vi "Periodic Tasks.vi"(8 "error in":errorcluster) -> ()   [LabVIEW 2015]
doc: "This VI runs in parallel to other tasks. It can contain as many user-defined periodic loops as you need. These can carry out PID or other sorts of timed response."
uses:
  LowGoalState.ctl
  SonarAction.ctl
  Example_Code/PressureSensor/PressureSensorAction.ctl
  RefnameEnum.ctl
  ServoAction.ctl
  TankDriveAction.ctl
  AutoAlignMode.ctl
  LEDSaction.ctl
  CatchAction.ctl
  CollectorWrapAction.ctl
  ShooterWrapperAction.ctl
  CollectorAction.ctl
  DoubleSolenoidAction.ctl
  SingleSolenoidAction.ctl
  <vilib>/Rock Robotics/SystemInterfaces/Utilities/FPGA_UtilitiesLED Source.ctl
  <vilib>/Rock Robotics/SystemInterfaces/Utilities/FPGA_UtilitiesLED State.ctl
  Robot Global Data.vi
  ArcadeDrivePieceWise.vi
  <vilib>/Rock Robotics/WPI/Compressor/WPI_CompressorGetSetRefNum.vi
  PassState.ctl
panel:
  in  "ShooterWait":i32=750
  in  "ShooterPassWait":i32
  in  "CutoffPressure":dbl=70.0
  out "LowGoalShotTimer":u32=50
  out "LowGoalShotIterations":i32=2744
  in  "PiecewiseCutoff":dbl=0.7 format="%#_13g"
  in  "ArcadeDeadzone":dbl=0.05 format="%#_13g"
  out "PassTimer":u32
  out "PassIterations":i32
  out "ServoTimer":u32
  out "ServoIterations":i32
  in  "HalfDriveScaler":dbl=0.7 min=0.0 max=1.0 step=0.05 format="%#_13g"
  out "ElevatedPassTimer":u32=50
  out "ElevatedPassIterations":i32=2744
  out "GroundPassTimer":u32=50
  out "GroundWrapperIterations":i32=2743
  out "PressureSensorTimer":u32
  out "PressureSensorIterations":i32
  out "AutoDistanceIterations":i32=6512
  out "AutoDistanceTimer":u32=20
  in  "Slowdown":dbl=12.0 format="%#_13g"
  in  "Brake":dbl=6.0 format="%#_13g"
  in  "DesiredDistance":dbl=144.0 format="%#_13g"
  out "CatcherWrapperIterations":i32=2744
  out "CatcherWrapperTimer":u32=50
  out "CollectorWrapperTimer":u32=50
  out "CollectorWrapperIterations":i32=2743
  out "ShooterWrapperIterations":i32=2667
  out "ShooterWrapperTimer":u32=50
  out "CollectorIterations":i32=2737
  out "ClapperIterations":i32=2743
  out "RollerPneumaticIterations":i32=2743
  out "RollerMotorIterations":i32=2742
  out "FiringCylinderIterations":i32=2745
  out "KickerIterations":i32=2744
  out "SonicShifterIterations":i32=2744
  out "TankDriveIterations":i32=6485
  out "Collector Timer":u32=50
  out "Clapper Timer":u32=50
  out "Roller Pneumatic Timer":u32=50
  out "Firing Cylinder Timer":u32=50
  out "Sonic Shifter Timer":u32=50
  out "Kicker Timer":u32=50
  out "Roller Motor Timer":u32=51
  out "Tank Drive Timer":u32=21
  # "ARCADE"
  # "CATCH"
  # "SHOOTER WRAP"
  # "SONIC SHIFTER"
  # "TANK DRIVE"
  # "KICKER"
  # "PRESSURE SENSOR"
  # "COLLECTOR WRAP"
  # "COLLECTOR ARM"
  # "ROLLER MOTOR"
  # "SERVO"
  # "FIRING CYLINDERS"
  # "AUTODISTANCE"
  # "ROLLER PNEUMATIC"
  # "CLAPPER"
  # "ELEVATED PASS"
  # "GROUND PASS"
  # "COMBINED PASS"
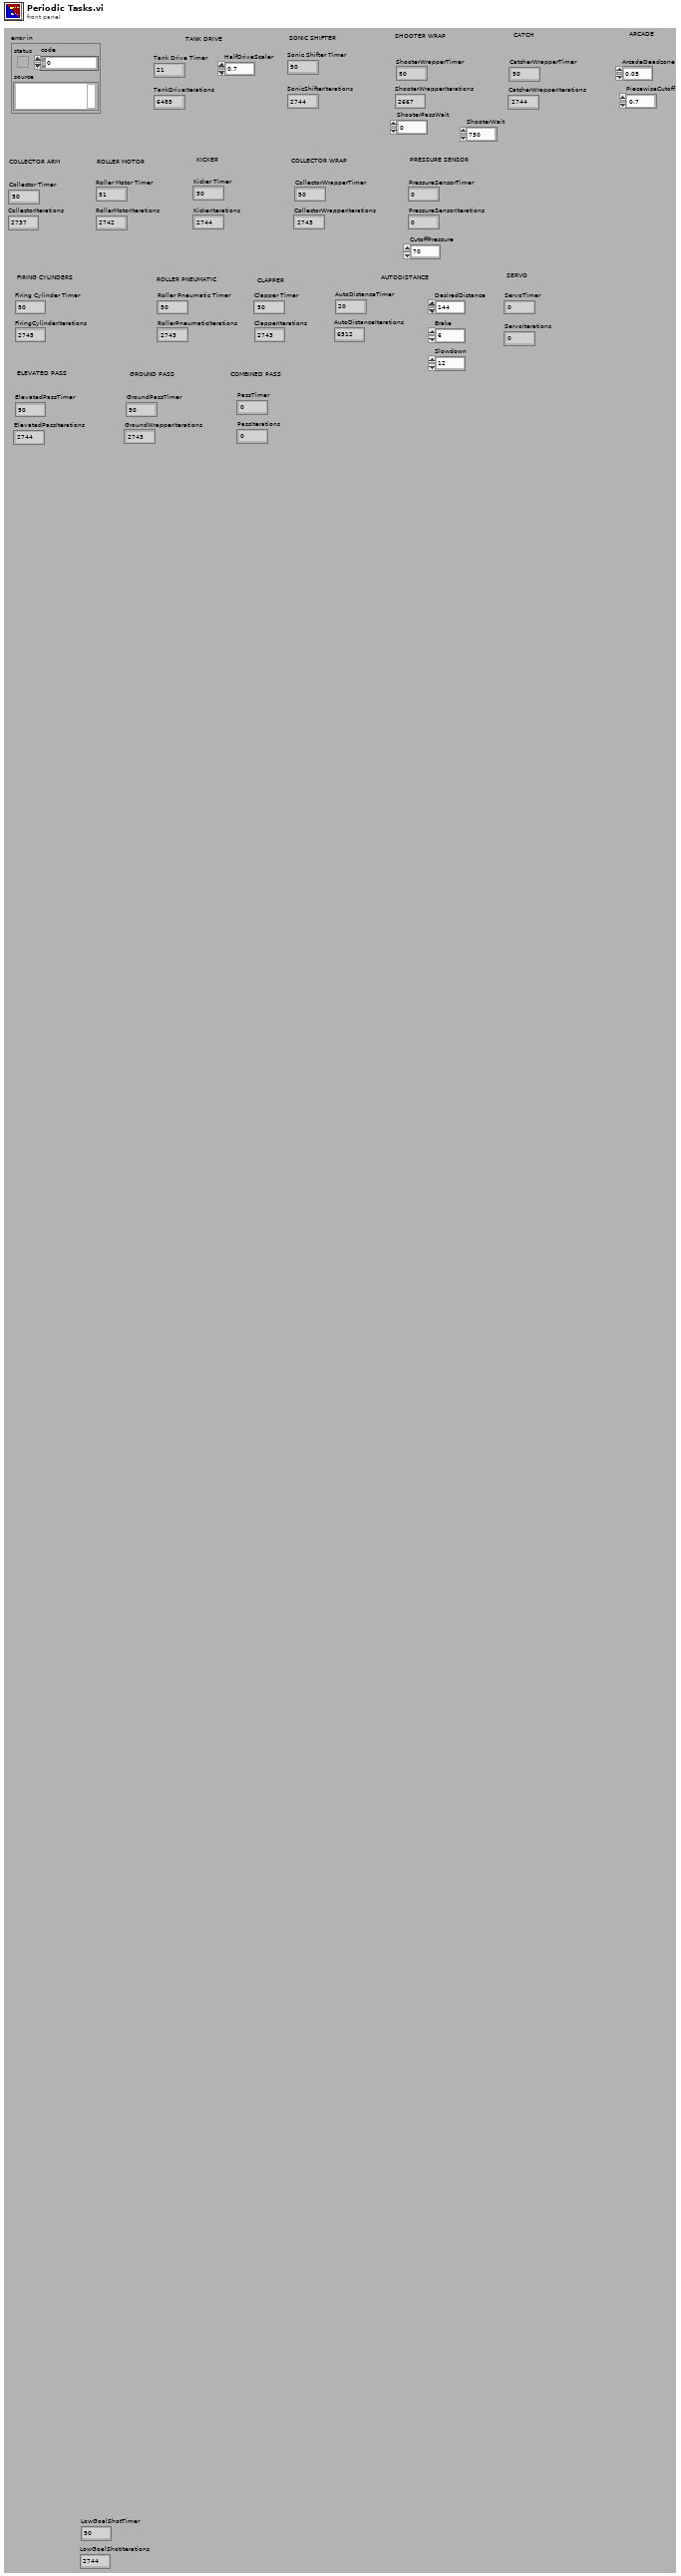
[diagram p1: front panel]
types:
  T1 = typedef "ShooterWrapperAction.ctl" = enum16{"Init", "CollectorDown", "CollectorUp"}
  T2 = typedef "CatchAction.ctl" = enum16{"Stop", "PreCatch", "Catch"}
  T3 = typedef "DoubleSolenoidAction.ctl" = enum16{"Init", "Middle", "In", "Out"}
  T4 = typedef "CollectorWrapAction.ctl" = enum16{"Stop", "PreCollect", "Collect"}
  T5 = typedef "SingleSolenoidAction.ctl" = enum16{"Init", "SetState", "Disable"}
  T6 = typedef "CollectorAction.ctl" = enum16{"Init", "Raise", "Lower", "Stop", "GetStatus"}
  T7 = typedef "FPGA_UtilitiesLED State.ctl" = enum16{"Off", "On", "Toggle"}
  T8 = typedef "FPGA_UtilitiesLED Source.ctl" = enum16{"User LED", "FPGA LED"}
  T9 = typedef "RefnameEnum.ctl" = enum16{"TankDrive", "Controller1", "Controller2", "SonicShifter", "Compressor"}
  T10 = typedef "WPI_CompressorDevRef.ctl" = cluster{"DevStatus":errorcluster, "DigitalInputDevRef":T11, "RelayDevRef":T14}
  T11 = typedef "WPI_DigitalInputDevRef.ctl" = cluster{"DevStatus":errorcluster, "DIO Channel":T12, "Digital Module":T13}
  T12 = typedef "FPGA_DIOChannel.ctl" = enum8{"DIO 1", "DIO 2", "DIO 3", "DIO 4", "DIO 5", "DIO 6", "DIO 7", "DIO 8", "DIO 9", "DIO 10", "DIO 11", "DIO 12", "DIO 13", "DIO 14", "Invalid"}
  T13 = typedef "FPGA_TypedefDigitalModule.ctl" = enum16{"Digital Module 1", "Digital Module 2"}
  T14 = typedef "WPI_RelayDevRef.ctl" = cluster{"DevStatus":errorcluster, "Relay Channel":T15, "Digital Module":T13, "Relay Direction":T16}
  T15 = typedef "FPGA_DIORelayChannel.ctl" = enum8{"Relay 1", "Relay 2", "Relay 3", "Relay 4", "Relay 5", "Relay 6", "Relay 7", "Relay 8", "Invalid"}
  T16 = typedef "WPI_RelayDirection.ctl" = enum16{"Both directions", "Forward only", "Reverse only"}
  T17 = typedef "RollerAction.ctl" = enum16{"Init", "Off", "Forward", "Reverse"}
  T18 = typedef "TankDriveAction.ctl" = enum16{"Init", "LinearDrive", "SetValue", "Disable"}
  T19 = typedef "SonarAction.ctl" = enum16{"Init", "ReadValue", "Disable"}
  T20 = typedef "AutoAlignMode.ctl" = enum16{"Fullspeed", "Linear"}
  T21 = typedef "PressureSensorAction.ctl" = enum16{"Init", "ReadValue", "Disable"}
  T22 = typedef "LEDSaction.ctl" = enum16{"Init", "10SecondsLeft", "LimitDown", "LimitUp", "CollectDown", "CollectUp", "NotHot", "Hot", "Shift", "RollBack", "RollFwd", "Shoot", "Distance Low", "DistanceHigh", "PressureLow", "PressureHigh"}
  T23 = typedef "PassState.ctl" = enum16{"Stop", "Pass"}
  T24 = typedef "ServoAction.ctl" = enum16{"Init", "SetAngle", "GetAngle", "Lower", "Raise", "Disable"}
  T25 = typedef "PassType.ctl" = enum16{"Ground", "Elevated"}
  T26 = typedef "LowGoalState.ctl" = enum16{"Stop", "Shoot"}
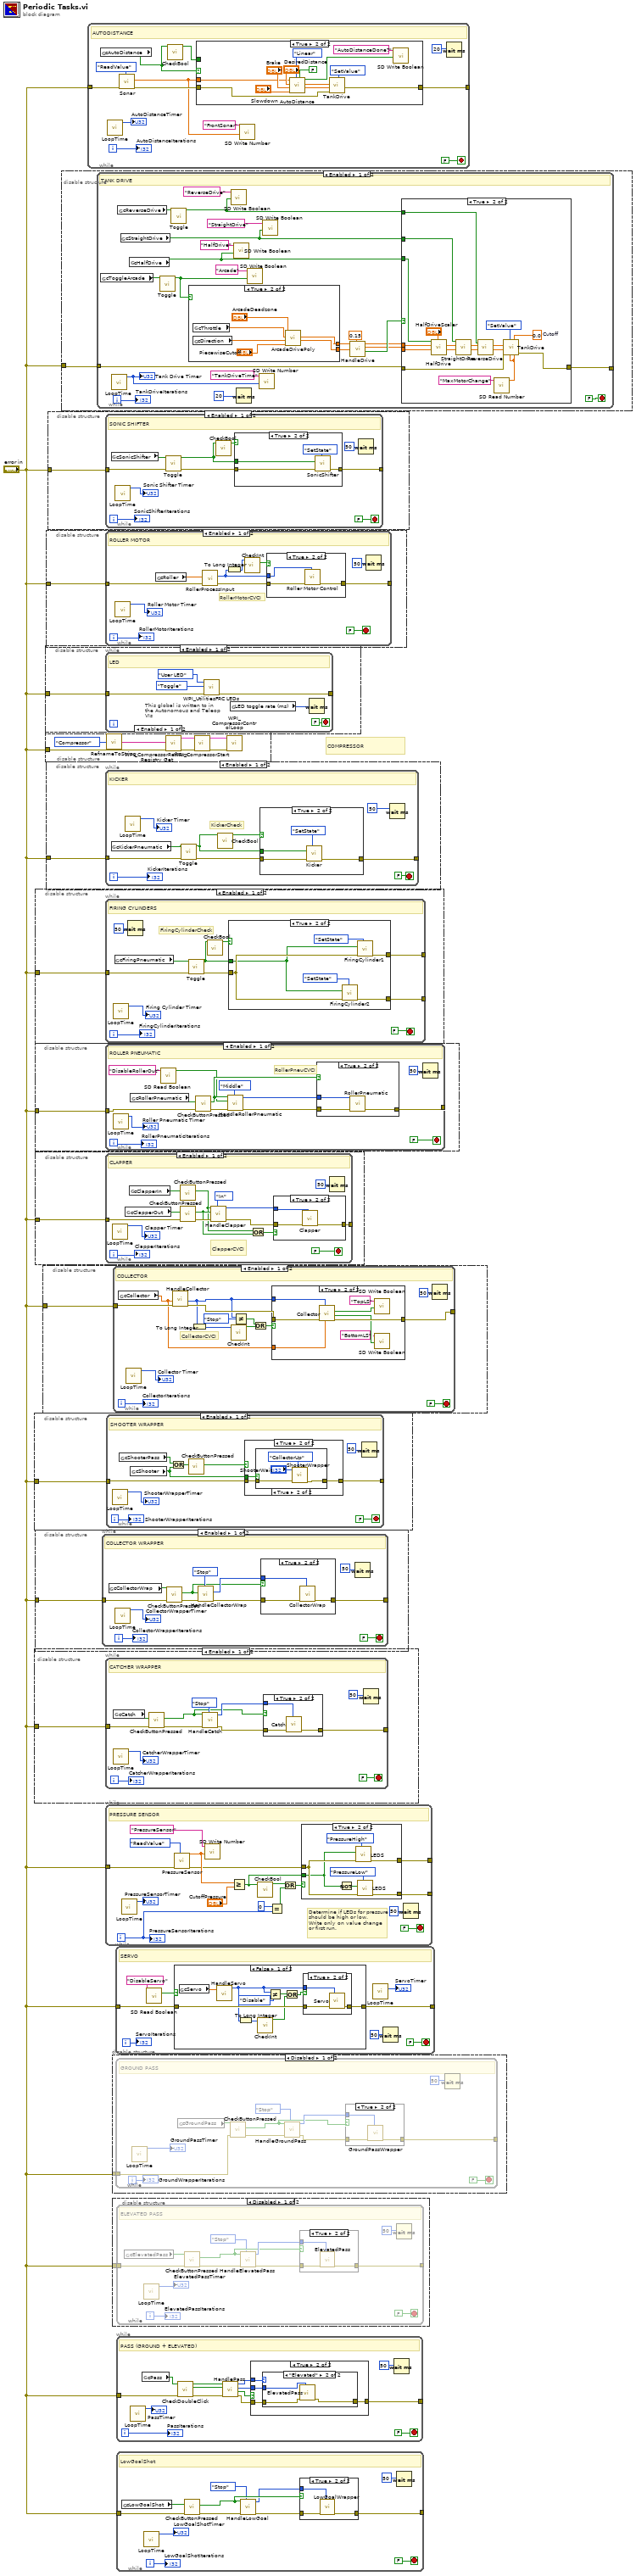
[diagram p0: block diagram]
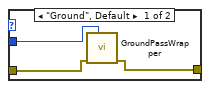
[diagram p4: hidden frame]
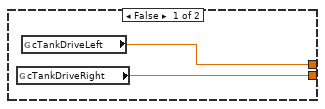
[diagram p11: hidden frame]
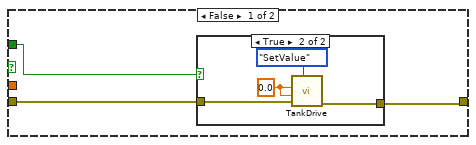
[diagram p14: hidden frame]
diagram:
  # "COMPRESSOR"
  n1 = disable-structure shown="Enabled" {
    disable-tunnel: "error in" -> [w2 _]
    frame Enabled {
      n2 = while {
        tunnel: w2 -> [w10]
        tunnel: [w9] -> _
        i -> [w8]
        stop <- FALSE stop-if-true
        # "SHOOTER WRAPPER"
        n3 = call "LoopTime.vi"() -> ("LoopTime"=→"ShooterWrapperTimer":u32)  [unwired: 11 in]
        n4 = global read "Robot Global Data.vi" "cShooterPass"() -> (w4:bool)
        n5 = global read "Robot Global Data.vi" "cShooter"() -> (w3:bool)
        n6 = Or(x=w4, y=w3) -> (x .or. y?=w5:bool)
        n7 = call "CheckButtonPressed.vi"("Button"=w5) -> ("Pressed?"=w6:bool)  [unwired: 9 in, 1 out]
        n8 = case shown="True" w6 {
          tunnel: w10 -> [w13 w16]
          tunnel: [w13 w15] -> w9
          tunnel: w3 -> [_ w14]
          frame False {
          }
          frame True {
            n9 = case shown="True" w14 {
              tunnel: w16 -> [w19 w24]
              tunnel: [w18 w23] -> w15
              frame False {
                n10 = call "ShooterWrapper.vi"("Action"=ShooterWrapperAction."CollectorUp", "error in"=w19, "ShooterWait"="ShooterPassWait") -> ("error out"=w18:errorcluster)  [unwired: 7 in]
              }
              frame True {
                n11 = call "ShooterWrapper.vi"("Action"=ShooterWrapperAction."CollectorUp", "error in"=w24, "ShooterWait"="ShooterWait") -> ("error out"=w23:errorcluster)  [unwired: 7 in]
              }
            }
          }
        }
        n12 = Wait (ms)(milliseconds to wait=u32 50) -> ()  [unwired: 1 out]
        "ShooterWrapperIterations" <- w8
      }
    }
    frame Disabled {
    }
  }
  n13 = disable-structure shown="Enabled" {
    disable-tunnel: "error in" -> [w25 _]
    frame Enabled {
      n14 = while {
        tunnel: w25 -> [w37]
        tunnel: [w35] -> _
        i -> [w33]
        stop <- FALSE stop-if-true
        # "CATCHER WRAPPER"
        n15 = call "LoopTime.vi"() -> ("LoopTime"=→"CatcherWrapperTimer":u32)  [unwired: 11 in]
        n16 = global read "Robot Global Data.vi" "cCatch"() -> (w36:bool)
        n17 = call "CheckButtonPressed.vi"("error in (no error)"=w37, "Button"=w36) -> ("error out"=w31:errorcluster, "Pressed?"=w26:bool)  [unwired: 8 in]
        n18 = call "HandleCatch.vi"("InitState"=CatchAction."Stop", "error in (no error)"=w31, "ButtonPressed?"=w26) -> ("error out"=w30:errorcluster, "State"=w29:T2)  [unwired: 7 in]
        n19 = case shown="True" w26 {
          tunnel: w30 -> [w38 w41]
          tunnel: [w38 w40] -> w35
          tunnel: w29 -> [_ w39]
          frame False {
          }
          frame True {
            n20 = call "Catch.vi"("Action"=w39, "error in (no error)"=w41) -> ("error out"=w40:errorcluster)  [unwired: 9 in]
          }
        }
        n21 = Wait (ms)(milliseconds to wait=u32 50) -> ()  [unwired: 1 out]
        "CatcherWrapperIterations" <- w33
      }
    }
    frame Disabled {
    }
  }
  n22 = disable-structure shown="Enabled" {
    disable-tunnel: "error in" -> [w42 _]
    frame Enabled {
      n23 = while {
        tunnel: w42 -> [w49]
        tunnel: [w51] -> _
        i -> [w50]
        stop <- FALSE stop-if-true
        # "RollerPneuCVCI"
        # "ROLLER PNEUMATIC"
        n24 = call "LoopTime.vi"() -> ("LoopTime"=→"Roller Pneumatic Timer":u32)  [unwired: 11 in]
        n25 = global read "Robot Global Data.vi" "cRollerPneumatic"() -> (w47:bool)
        n26 = call <vilib>:"SD Read Boolean.vi"("Name"="DisableRollerOut") -> ("Boolean"=w43:bool)  [unwired: 8 in, 2 out]
        n27 = call "CheckButtonPressed.vi"("error in (no error)"=w49, "Button"=w47) -> ("error out"=w48:errorcluster, "Pressed?"=w45:bool)  [unwired: 8 in]
        n28 = call "HandleRollerPneumatic.vi"("InitState"=DoubleSolenoidAction."Middle", "error in (no error)"=w48, "DisableOut?"=w43, "ButtonPressed?"=w45) -> ("error out"=w52:errorcluster, "State"=w53:T3)  [unwired: 6 in]
        n29 = case shown="True" w45 {
          tunnel: w53 -> [_ w60]
          tunnel: w52 -> [w57 w59]
          tunnel: [w57 w58] -> w51
          frame False {
          }
          frame True {
            n30 = call "RollerPneumatic.vi"("State"=w60, "Error in"=w59) -> ("Error out"=w58:errorcluster)  [unwired: 9 in]
          }
        }
        n31 = Wait (ms)(milliseconds to wait=u32 50) -> ()  [unwired: 1 out]
        "RollerPneumaticIterations" <- w50
      }
    }
    frame Disabled {
    }
  }
  n32 = disable-structure shown="Enabled" {
    disable-tunnel: "error in" -> [w61 _]
    frame Enabled {
      n33 = while {
        tunnel: w61 -> [w69]
        tunnel: [w71] -> _
        i -> [w70]
        stop <- FALSE stop-if-true
        # "COLLECTOR WRAPPER"
        n34 = global read "Robot Global Data.vi" "cCollectorWrap"() -> (w68:bool)
        n35 = call "LoopTime.vi"() -> ("LoopTime"=→"CollectorWrapperTimer":u32)  [unwired: 11 in]
        n36 = call "CheckButtonPressed.vi"("error in (no error)"=w69, "Button"=w68) -> ("error out"=w67:errorcluster, "Pressed?"=w62:bool)  [unwired: 8 in]
        n37 = call "HandleCollectorWrap.vi"("InitState"=CollectorWrapAction."Stop", "error in (no error)"=w67, "ButtonPressed?"=w62) -> ("error out"=w65:errorcluster, "State"=w64:T4)  [unwired: 7 in]
        n38 = case shown="True" w62 {
          tunnel: [w74 w77] -> w71
          tunnel: w65 -> [w74 w76]
          tunnel: w64 -> [_ w75]
          frame False {
          }
          frame True {
            n39 = call "CollectorWrap.vi"("Action"=w75, "error in"=w76) -> ("error out"=w77:errorcluster)  [unwired: 9 in]
          }
        }
        n40 = Wait (ms)(milliseconds to wait=u32 50) -> ()  [unwired: 1 out]
        "CollectorWrapperIterations" <- w70
      }
    }
    frame Disabled {
    }
  }
  n41 = disable-structure shown="Enabled" {
    disable-tunnel: "error in" -> [w78 _]
    frame Enabled {
      n42 = while {
        tunnel: w78 -> [w84]
        tunnel: [w87] -> _
        tunnel: [w86] -> _
        i -> [w80]
        stop <- FALSE stop-if-true
        # "FiringCylinderCheck"
        # "FIRING CYLINDERS"
        n43 = call "LoopTime.vi"() -> ("LoopTime"=→"Firing Cylinder Timer":u32)  [unwired: 11 in]
        n44 = global read "Robot Global Data.vi" "cFiringPneumatic"() -> (w85:bool)
        n45 = Wait (ms)(milliseconds to wait=u32 50) -> ()  [unwired: 1 out]
        n46 = call "Toggle.vi"("error in"=w84, "RawInput"=w85) -> ("error out"=w83:errorcluster, "ToggleState"=w81:bool)  [unwired: 8 in]
        n47 = call "CheckBool.vi"("Input Boolean"=w81) -> ("Boolean Changed?"=w82:bool)  [unwired: 10 in]
        n48 = case shown="True" w82 {
          tunnel: w83 -> [w90 w92]
          tunnel: [w90 w94] -> w87
          tunnel: [w90 w93] -> w86
          tunnel: w81 -> [_ w91]
          frame False {
          }
          frame True {
            n49 = call "FiringCylinder2.vi"("Action"=SingleSolenoidAction."SetState", "error in (no error)"=w92, "Actuate?"=w91) -> ("error out"=w93:errorcluster)  [unwired: 8 in]
            n50 = call "FiringCylinder1.vi"("Action"=SingleSolenoidAction."SetState", "error in (no error)"=w92, "Actuate?"=w91) -> ("error out"=w94:errorcluster)  [unwired: 8 in]
          }
        }
        "FiringCylinderIterations" <- w80
      }
    }
    frame Disabled {
    }
  }
  n51 = disable-structure shown="Enabled" {
    disable-tunnel: "error in" -> [w97 _]
    frame Enabled {
      n52 = while {
        tunnel: w97 -> [w106]
        tunnel: [w109] -> _
        i -> [w107]
        stop <- FALSE stop-if-true
        # "ClapperCVCI"
        # "CLAPPER"
        n53 = call "LoopTime.vi"() -> ("LoopTime"=→"Clapper Timer":u32)  [unwired: 11 in]
        n54 = global read "Robot Global Data.vi" "cClapperOut"() -> (w103:bool)
        n55 = global read "Robot Global Data.vi" "cClapperIn"() -> (w102:bool)
        n56 = call "CheckButtonPressed.vi"("Button"=w102) -> ("Pressed?"=w98:bool)  [unwired: 9 in, 1 out]
        n57 = call "CheckButtonPressed.vi"("error in (no error)"=w106, "Button"=w103) -> ("error out"=w105:errorcluster, "Pressed?"=w99:bool)  [unwired: 8 in]
        n58 = call "HandleClapper.vi"("InitState"=DoubleSolenoidAction."In", "error in (no error)"=w105, "ClapperOut"=w99, "ClapperIn"=w98) -> ("error out"=w110:errorcluster, "State"=w108:T3)  [unwired: 6 in]
        n59 = Or(x=w98, y=w99) -> (x .or. y?=w100:bool)
        n60 = case shown="True" w100 {
          tunnel: w108 -> [_ w116]
          tunnel: w110 -> [w113 w115]
          tunnel: [w113 w114] -> w109
          frame False {
          }
          frame True {
            n61 = call "Clapper.vi"("State"=w116, "Error in"=w115) -> ("Error out"=w114:errorcluster)  [unwired: 9 in]
          }
        }
        n62 = Wait (ms)(milliseconds to wait=u32 50) -> ()  [unwired: 1 out]
        "ClapperIterations" <- w107
      }
    }
    frame Disabled {
    }
  }
  n63 = disable-structure shown="Enabled" {
    disable-tunnel: "error in" -> [w117 _]
    frame Enabled {
      n64 = while {
        tunnel: w117 -> [w130]
        tunnel: [w126] -> _
        i -> [w125]
        stop <- FALSE stop-if-true
        # "CollectorCVCI"
        # "COLLECTOR"
        n65 = global read "Robot Global Data.vi" "cCollector"() -> (w124:dbl)
        n66 = call "LoopTime.vi"() -> ("LoopTime"=→"Collector Timer":u32)  [unwired: 11 in]
        n67 = call "HandleCollector.vi"("error in"=w130, "JoystickValue"=w124) -> ("error out"=w127:errorcluster, "CollectorEnum Input"=w122:T6)  [unwired: 8 in]
        n68 = To Long Integer(number=w122) -> (32bit integer=w128:i32)
        n69 = call "CheckInt.vi"("Integer"=w128) -> ("Changed?"=w118:bool)  [unwired: 10 in]
        n70 = Not Equal?(x=w122, y=CollectorAction."Stop") -> (x != y?=w119:bool)
        n71 = Or(x=w119, y=w118) -> (x .or. y?=w120:bool)
        n72 = case shown="True" w120 {
          tunnel: w122 -> [_ w140]
          tunnel: w127 -> [w132 w139]
          tunnel: [w132 w138] -> w126
          tunnel: w124 -> [_ w133]
          frame False {
          }
          frame True {
            n73 = call "Collector.vi"("MotorSpeed"=w133, "Action"=w140, "Error in"=w139) -> ("Error out"=w138:errorcluster, "Lower Triggered?"=w136:bool, "Upper Triggered?"=w137:bool)  [unwired: 6 in]
            n74 = call <vilib>:"SD Write Boolean.vi"("Boolean"=w137, "Name"="TopLS") -> ()  [unwired: 8 in, 2 out]
            n75 = call <vilib>:"SD Write Boolean.vi"("Boolean"=w136, "Name"="BottomLS") -> ()  [unwired: 8 in, 2 out]
          }
        }
        n76 = Wait (ms)(milliseconds to wait=u32 50) -> ()  [unwired: 1 out]
        "CollectorIterations" <- w125
      }
    }
    frame Disabled {
    }
  }
  n77 = disable-structure shown="Enabled" {
    disable-tunnel: "error in" -> [w141 _]
    frame Enabled {
      n78 = while {
        tunnel: w141 -> [w143]
        tunnel: [w142] -> _
        stop <- FALSE stop-if-true
        # "This global is written to in the Autonomous and Teleop VIs"
        # "LED"
        n79 = call <vilib>:"WPI_UtilitiesFRC LEDs.vi"("error in (no error)"=w143, "State"=FPGA_UtilitiesLED_State."Toggle", "LED Type"=FPGA_UtilitiesLED_Source."User LED") -> ("error out"=w142:errorcluster)  [unwired: 8 out]
        n80 = global read "Robot Global Data.vi" "LED toggle rate (ms)"() -> (w144:u32)
        n81 = Wait (ms)(milliseconds to wait=w144) -> ()  [unwired: 1 out]
      }
    }
    frame Disabled {
    }
  }
  n82 = disable-structure shown="Enabled" {
    disable-tunnel: "error in" -> [w154 _]
    frame Enabled {
      n83 = call "RefnameToString.vi"("Enum"=RefnameEnum."Compressor") -> ("Refname"=w153:string)
      n84 = call <vilib>:"WPI_CompressorRefNum Registry Get.vi"("error in (no error)"=w154, "refnum name"=w153) -> ("error out"=w149:errorcluster, "CompressorDevRef"=w151:T10)  [unwired: 8 in]
      n85 = call <vilib>:"WPI_CompressorStart.vi"("error in (no error)"=w149, "CompressorDevRef"=w151) -> ("error out"=w148:errorcluster, "CompressorDevRef"=w150:T10)  [unwired: 8 in]
      n86 = call <vilib>:"WPI_CompressorControlLoop.vi"("error in (no error)"=w148, "CompressorDevRef"=w150) -> ()  [unwired: 10 in]
    }
    frame Disabled {
    }
  }
  n87 = disable-structure shown="Enabled" {
    disable-tunnel: "error in" -> [w155 _]
    frame Enabled {
      n88 = while {
        tunnel: w155 -> [w164]
        tunnel: [w159] -> _
        i -> [w157]
        stop <- FALSE stop-if-true
        # "RollerMotorCVCI"
        # "ROLLER MOTOR"
        n89 = call "LoopTime.vi"() -> ("LoopTime"=→"Roller Motor Timer":u32)  [unwired: 11 in]
        n90 = global read "Robot Global Data.vi" "cRoller"() -> (w163:dbl)
        n91 = call "RollerProcessInput.vi"("error in"=w164, "JoystickValue"=w163) -> ("error out"=w160:errorcluster, "StateOut"=w158:T17)  [unwired: 8 in]
        n92 = To Long Integer(number=w158) -> (32bit integer=w162:i32)
        n93 = call "CheckInt.vi"("Integer"=w162) -> ("Changed?"=w161:bool)  [unwired: 10 in]
        n94 = case shown="True" w161 {
          tunnel: w158 -> [_ w170]
          tunnel: w160 -> [w167 w169]
          tunnel: [w167 w168] -> w159
          frame False {
          }
          frame True {
            n95 = call "Roller Motor Control.vi"("Action"=w170, "Error in"=w169) -> ("Error out"=w168:errorcluster)  [unwired: 9 in]
          }
        }
        n96 = Wait (ms)(milliseconds to wait=u32 50) -> ()  [unwired: 1 out]
        "RollerMotorIterations" <- w157
      }
    }
    frame Disabled {
    }
  }
  n97 = disable-structure shown="Enabled" {
    disable-tunnel: "error in" -> [w171 _]
    frame Enabled {
      n98 = while {
        tunnel: w171 -> [w178]
        tunnel: [w179] -> _
        i -> [w173]
        stop <- FALSE stop-if-true
        # "KickerCheck"
        # "KICKER"
        n99 = global read "Robot Global Data.vi" "cKickerPneumatic"() -> (w176:bool)
        n100 = call "LoopTime.vi"() -> ("LoopTime"=→"Kicker Timer":u32)  [unwired: 11 in]
        n101 = call "Toggle.vi"("error in"=w178, "RawInput"=w176) -> ("error out"=w177:errorcluster, "ToggleState"=w174:bool)  [unwired: 8 in]
        n102 = call "CheckBool.vi"("Input Boolean"=w174) -> ("Boolean Changed?"=w175:bool)  [unwired: 10 in]
        n103 = case shown="True" w175 {
          tunnel: w177 -> [w182 w184]
          tunnel: [w182 w185] -> w179
          tunnel: w174 -> [_ w183]
          frame False {
          }
          frame True {
            n104 = call "Kicker.vi"("Action"=SingleSolenoidAction."SetState", "error in (no error)"=w184, "Actuate?"=w183) -> ("error out"=w185:errorcluster)  [unwired: 8 in]
          }
        }
        n105 = Wait (ms)(milliseconds to wait=u32 50) -> ()  [unwired: 1 out]
        "KickerIterations" <- w173
      }
    }
    frame Disabled {
    }
  }
  n106 = disable-structure shown="Enabled" {
    disable-tunnel: "error in" -> [w187 _]
    frame Enabled {
      n107 = while {
        tunnel: w187 -> [w193]
        tunnel: [w195] -> _
        i -> [w190]
        stop <- FALSE stop-if-true
        # "SONIC SHIFTER"
        n108 = global read "Robot Global Data.vi" "cSonicShifter"() -> (w194:bool)
        n109 = call "LoopTime.vi"() -> ("LoopTime"=→"Sonic Shifter Timer":u32)  [unwired: 11 in]
        n110 = call "Toggle.vi"("error in"=w193, "RawInput"=w194) -> ("error out"=w192:errorcluster, "ToggleState"=w189:bool)  [unwired: 8 in]
        n111 = call "CheckBool.vi"("Input Boolean"=w189) -> ("Boolean Changed?"=w191:bool)  [unwired: 10 in]
        n112 = case shown="True" w191 {
          tunnel: [w198 w201] -> w195
          tunnel: w192 -> [w198 w200]
          tunnel: w189 -> [_ w199]
          frame False {
          }
          frame True {
            n113 = call "SonicShifter.vi"("Action"=SingleSolenoidAction."SetState" ("Mode"), "error in (no error)"=w200, "Actuate?"=w199) -> ("error out"=w201:errorcluster)  [unwired: 8 in]
          }
        }
        n114 = Wait (ms)(milliseconds to wait=u32 50) -> ()  [unwired: 1 out]
        "SonicShifterIterations" <- w190
      }
    }
    frame Disabled {
    }
  }
  n115 = disable-structure shown="Enabled" {
    disable-tunnel: "error in" -> [w203 _]
    frame Enabled {
      n116 = while {
        tunnel: w203 -> [w217]
        tunnel: [w222] -> _
        i -> [w219]
        stop <- FALSE stop-if-true
        # "TANK DRIVE"
        n117 = global read "Robot Global Data.vi" "cToggleArcade"() -> (w208:bool)
        n118 = call "LoopTime.vi"() -> ("LoopTime"=w215:u32)  [unwired: 11 in]
        "Tank Drive Timer" <- w215
        n119 = global read "Robot Global Data.vi" "cReverseDrive"() -> (w218:bool)
        n120 = global read "Robot Global Data.vi" "cStraightDrive"() -> (w210:bool)
        n121 = global read "Robot Global Data.vi" "cHalfDrive"() -> (w209:bool)
        n122 = call "Toggle.vi"("RawInput"=w208) -> ("ToggleState"=w206:bool)  [unwired: 9 in, 1 out]
        n123 = call "Toggle.vi"("RawInput"=w218) -> ("ToggleState"=w216:bool)  [unwired: 9 in, 1 out]
        n124 = case shown="True" w206 {
          tunnel: [w228 w230] -> w205
          tunnel: [w227 w229] -> w204
          frame False {
            n125 = global read "Robot Global Data.vi" "cTankDriveRight"() -> (w227:dbl)
            n126 = global read "Robot Global Data.vi" "cTankDriveLeft"() -> (w228:dbl)
          }
          frame True {
            n127 = global read "Robot Global Data.vi" "cDirection"() -> (w233:dbl)
            n128 = global read "Robot Global Data.vi" "cThrottle"() -> (w234:dbl)
            n129 = call-poly "ArcadeDrivePoly.vi"("Cutoff"="PiecewiseCutoff", "Direction"=w233, "Throttle"=w234, "Deadzone"="ArcadeDeadzone") -> ("DriveRight"=w229:dbl, "DriveLeft"=w230:dbl)  [unwired: 6 in]
          }
        }
        n130 = call <vilib>:"SD Write Boolean.vi"("Boolean"=w216, "Name"="ReverseDrive") -> ()  [unwired: 8 in, 2 out]
        n131 = call <vilib>:"SD Write Boolean.vi"("Boolean"=w209, "Name"="HalfDrive") -> ()  [unwired: 8 in, 2 out]
        n132 = Wait (ms)(milliseconds to wait=u32 20) -> ()  [unwired: 1 out]
        n133 = call <vilib>:"SD Write Boolean.vi"("Boolean"=w206, "Name"="Arcade") -> ()  [unwired: 8 in, 2 out]
        n134 = call <vilib>:"SD Write Number.vi"("Numeric"=w215, "Name"="TankDriveTime") -> ()  [unwired: 8 in, 2 out]
        n135 = call <vilib>:"SD Write Boolean.vi"("Boolean"=w210, "Name"="StraightDrive") -> ()  [unwired: 8 in, 2 out]
        n136 = call "HandleDrive.vi"("Deadzone"=0.15, "RightMotor"=w204, "LeftMotor"=w205) -> ("Enqueue?"=w225:bool, "RightMotor"=w223:dbl, "LeftMotor"=w224:dbl)  [unwired: 6 in]
        n137 = case shown="True" w225 {
          tunnel: w224 -> [_ w245]
          tunnel: w223 -> [_ w244]
          tunnel: [w235 w243] -> w222
          tunnel: w217 -> [w235 w242]
          tunnel: w216 -> [_ w240]
          tunnel: w209 -> [_ w239]
          tunnel: w210 -> [_ w238]
          frame False {
          }
          frame True {
            w252 = 0.0  # Cutoff
            n138 = call "HalfDrive.vi"("Scaler"="HalfDriveScaler", "RightDrive in"=w244, "LeftDrive in"=w245, "HalfDrive"=w239) -> ("RightDrive out"=w251:dbl, "LeftDrive out"=w250:dbl)  [unwired: 6 in]
            n139 = call "StraightDrive.vi"("RightDrive in"=w251, "LeftDrive in"=w250, "StraightDrive"=w238) -> ("RightDrive out"=w248:dbl, "LeftDrive out"=w249:dbl)  [unwired: 7 in]
            n140 = call "ReverseDrive.vi"("cReverseDrive"=w240, "Right"=w248, "Left"=w249) -> ("Right"=w246:dbl, "Left"=w247:dbl)  [unwired: 7 in]
            n141 = call <vilib>:"SD Read Number.vi"("Name"="MaxMotorChange") -> ("Numeric"=w236:dbl)  [unwired: 8 in, 2 out]
            n142 = call "TankDrive.vi"("MaxMotorChangeForward"=w236, "Cutoff"=w252, "MaxMotorChangeBackwrad"=w236, "DriveAction"=TankDriveAction."SetValue", "error in (no error)"=w242, "RightDesired"=w246, "LeftDesired"=w247) -> ("error out"=w243:errorcluster)  [unwired: 3 in, 1 out]
          }
        }
        "TankDriveIterations" <- w219
      }
    }
    frame Disabled {
    }
  }
  n143 = while {
    tunnel: "error in" -> [w258]
    tunnel: [w265] -> _
    i -> [w263]
    stop <- FALSE stop-if-true
    # "AUTODISTANCE"
    n144 = global read "Robot Global Data.vi" "cAutoDistance"() -> (w261:bool)
    n145 = call "LoopTime.vi"() -> ("LoopTime"=→"AutoDistanceTimer":u32)  [unwired: 11 in]
    n146 = call "Sonar.vi"("Action"=SonarAction."ReadValue", "error in (no error)"=w258) -> ("error out"=w257:errorcluster, "distance"=w255:dbl)  [unwired: 8 in]
    n147 = call "CheckBool.vi"("Input Boolean"=w261) -> ("Boolean Changed?"=w260:bool)  [unwired: 10 in]
    n148 = case shown="True" w261 {
      tunnel: w257 -> [w268 w276]
      tunnel: [w267 w281] -> w265
      tunnel: w260 -> [w266 _]
      tunnel: w255 -> [_ w275]
      frame False {
        n149 = case shown="True" w266 {
          tunnel: w268 -> [w269 w273]
          tunnel: [w269 w272] -> w267
          frame False {
          }
          frame True {
            w271 = 0.0 ("LeftDesired")
            n150 = call "TankDrive.vi"("DriveAction"=TankDriveAction."SetValue", "error in (no error)"=w273, "RightDesired"=w271, "LeftDesired"=w271) -> ("error out"=w272:errorcluster)  [unwired: 6 in, 1 out]
          }
        }
      }
      frame True {
        n151 = call "AutoDistance.vi"("Auto"=FALSE, "Mode"=AutoAlignMode."Linear", "Slowdown"="Slowdown", "Brake"="Brake", "DesiredDistance"="DesiredDistance", "CurrentDistance"=w275) -> ("TankDriveRight"=w277:dbl, "TankDriveLeft"=w278:dbl, "Finished"=w280:bool)  [unwired: 3 in]
        n152 = call "TankDrive.vi"("DriveAction"=TankDriveAction."SetValue", "error in (no error)"=w276, "RightDesired"=w277, "LeftDesired"=w278) -> ("error out"=w281:errorcluster)  [unwired: 6 in, 1 out]
        n153 = call <vilib>:"SD Write Boolean.vi"("Boolean"=w280, "Name"="AutoDistanceDone?") -> ()  [unwired: 8 in, 2 out]
      }
    }
    n154 = call <vilib>:"SD Write Number.vi"("Numeric"=w255, "Name"="FrontSonar") -> ()  [unwired: 8 in, 2 out]
    n155 = Wait (ms)(milliseconds to wait=u32 20) -> ()  [unwired: 1 out]
    "AutoDistanceIterations" <- w263
  }
  n156 = while {
    tunnel: "error in" -> [w302]
    tunnel: [w293] -> _
    tunnel: [w292] -> _
    i -> [w291]
    stop <- FALSE stop-if-true
    # "Determine if LEDs for pressure\nshould be high or low.\nWrite only on value change\nor first run."
    # "PRESSURE SENSOR"
    n157 = call "LoopTime.vi"() -> ("LoopTime"=→"PressureSensorTimer":u32)  [unwired: 11 in]
    n158 = call "PressureSensor.vi"("Action"=PressureSensorAction."ReadValue", "error in (no error)"=w302) -> ("error out"=w295:errorcluster, "Pressure"=w297:dbl)  [unwired: 8 in]
    n159 = call <vilib>:"SD Write Number.vi"("Numeric"=w297, "Name"="PressureSensor") -> ()  [unwired: 8 in, 2 out]
    n160 = Greater Or Equal?(x=w297, y="CutoffPressure") -> (x >= y?=w294:bool)
    n161 = call "CheckBool.vi"("Input Boolean"=w294) -> ("Boolean Changed?"=w288:bool)  [unwired: 10 in]
    n162 = Equal?(x=0, y=w291) -> (x = y?=w289:bool)
    n163 = Or(x=w288, y=w289) -> (x .or. y?=w287:bool)
    n164 = case shown="True" w287 {
      tunnel: w295 -> [w304 w308]
      tunnel: [w304 w310] -> w293
      tunnel: w294 -> [_ w306]
      tunnel: [w304 w305] -> w292
      frame False {
      }
      frame True {
        n165 = Not(x=w306) -> (.not. x?=w307:bool)
        n166 = call "LEDS.vi"("Action"=LEDSaction."PressureHigh", "error in"=w308, "On/Off"=w306) -> ("error out"=w310:errorcluster)  [unwired: 8 in]
        n167 = call "LEDS.vi"("Action"=LEDSaction."PressureLow", "error in"=w308, "On/Off"=w307) -> ("error out"=w305:errorcluster)  [unwired: 8 in]
      }
    }
    n168 = Wait (ms)(milliseconds to wait=u32 50) -> ()  [unwired: 1 out]
    "PressureSensorIterations" <- w291
  }
  n169 = disable-structure shown="Disabled" {
    disable-tunnel: "error in" -> [w312 _]
    frame Disabled {
      n170 = while {
        tunnel: w312 -> [w320]
        tunnel: [w319] -> _
        i -> [w318]
        stop <- FALSE stop-if-true
        # "GROUND PASS"
        n171 = call "LoopTime.vi"() -> ("LoopTime"=→"GroundPassTimer":u32)  [unwired: 11 in]
        n172 = global read "Robot Global Data.vi" "cGroundPass"() -> (w315:bool)
        n173 = call "CheckButtonPressed.vi"("error in (no error)"=w320, "Button"=w315) -> ("error out"=w322:errorcluster, "Pressed?"=w314:bool)  [unwired: 8 in]
        n174 = call "HandleGroundPass.vi"("InitState"=PassState."Stop", "error in"=w322, "Toggle?"=w314) -> ("error out"=w321:errorcluster, "State"=w317:T23)  [unwired: 7 in]
        n175 = case shown="True" w314 {
          tunnel: w321 -> [w325 w328]
          tunnel: [w325 w327] -> w319
          tunnel: w317 -> [_ w326]
          frame False {
          }
          frame True {
            n176 = call "GroundPassWrapper.vi"("State"=w326, "error in"=w328) -> ("error out"=w327:errorcluster)  [unwired: 9 in]
          }
        }
        n177 = Wait (ms)(milliseconds to wait=u32 50) -> ()  [unwired: 1 out]
        "GroundWrapperIterations" <- w318
      }
    }
    frame Enabled {
    }
  }
  n178 = disable-structure shown="Disabled" {
    disable-tunnel: "error in" -> [w329 _]
    frame Disabled {
      n179 = while {
        tunnel: [w341] -> _
        tunnel: w329 -> [w334]
        i -> [w339]
        stop <- FALSE stop-if-true
        # "ELEVATED PASS"
        n180 = global read "Robot Global Data.vi" "cElevatedPass"() -> (w332:bool)
        n181 = call "LoopTime.vi"() -> ("LoopTime"=→"ElevatedPassTimer":u32)  [unwired: 11 in]
        n182 = call "CheckButtonPressed.vi"("error in (no error)"=w334, "Button"=w332) -> ("error out"=w337:errorcluster, "Pressed?"=w331:bool)  [unwired: 8 in]
        n183 = call "HandleElevatedPass.vi"("InitState"=PassState."Stop", "error in (no error)"=w337, "Toggle?"=w331) -> ("error out"=w336:errorcluster, "PassState"=w335:T23)  [unwired: 7 in]
        n184 = case shown="True" w331 {
          tunnel: w336 -> [w342 w345]
          tunnel: [w342 w344] -> w341
          tunnel: w335 -> [_ w343]
          frame False {
          }
          frame True {
            n185 = call "ElevatedPass.vi"("PassState"=w343, "error in (no error)"=w345) -> ("error out"=w344:errorcluster)  [unwired: 9 in]
          }
        }
        n186 = Wait (ms)(milliseconds to wait=u32 50) -> ()  [unwired: 1 out]
        "ElevatedPassIterations" <- w339
      }
    }
    frame Enabled {
    }
  }
  n187 = while {
    tunnel: [w352] -> _
    tunnel: "error in" -> [w350]
    i -> [w348]
    stop <- FALSE stop-if-true
    # "SERVO"
    n188 = call <vilib>:"SD Read Boolean.vi"("Name"="DisableServo") -> ("Boolean"=w347:bool)  [unwired: 8 in, 2 out]
    n189 = case shown="False" w347 {
      tunnel: [w362 w367] -> w352
      tunnel: w350 -> [w361 w367]
      frame False {
        n190 = global read "Robot Global Data.vi" "cServo"() -> (w360:dbl)
        n191 = call "HandleServo.vi"("DPadValue"=w360) -> ("Action"=w358:T24)  [unwired: 10 in]
        n192 = To Long Integer(number=w358) -> (32bit integer=w359:i32)
        n193 = call "CheckInt.vi"("Integer"=w359) -> ("Changed?"=w354:bool)  [unwired: 10 in]
        n194 = Not Equal?(x=w358, y=ServoAction."Disable") -> (x != y?=w355:bool)
        n195 = Or(x=w355, y=w354) -> (x .or. y?=w356:bool)
        n196 = case shown="True" w356 {
          tunnel: [w363 w366] -> w362
          tunnel: w361 -> [w363 w365]
          tunnel: w358 -> [_ w364]
          frame False {
          }
          frame True {
            n197 = call "Servo.vi"("Action"=w364, "error in (no error)"=w365) -> ("error out"=w366:errorcluster)  [unwired: 8 in, 1 out]
          }
        }
      }
      frame True {
      }
    }
    n198 = call "LoopTime.vi"() -> ("LoopTime"=→"ServoTimer":u32)  [unwired: 11 in]
    n199 = Wait (ms)(milliseconds to wait=u32 50) -> ()  [unwired: 1 out]
    "ServoIterations" <- w348
  }
  n200 = while {
    tunnel: "error in" -> [w377]
    tunnel: [w371] -> _
    i -> [w370]
    stop <- FALSE stop-if-true
    # "PASS (GROUND + ELEVATED)"
    n201 = call "LoopTime.vi"() -> ("LoopTime"=→"PassTimer":u32)  [unwired: 11 in]
    n202 = global read "Robot Global Data.vi" "cPass"() -> (w378:bool)
    n203 = call "CheckDoubleClick.vi"("error in (no error)"=w377, "cPass"=w378) -> ("error out"=w376:errorcluster, "Perform?"=w379:bool, "Double Click?"=w380:bool)  [unwired: 7 in]
    n204 = call "HandlePass.vi"("error in (no error)"=w376, "Perform?"=w379, "DoubleClick?"=w380) -> ("error out"=w372:errorcluster, "Call?"=w375:bool, "PassState"=w373:T23, "PassType"=w374:T25)  [unwired: 5 in]
    n205 = case shown="True" w375 {
      tunnel: w374 -> [_ w386]
      tunnel: w373 -> [_ w385]
      tunnel: w372 -> [w382 w384]
      tunnel: [w382 w383] -> w371
      frame False {
      }
      frame True {
        n206 = case shown="\"Elevated\"" w386 {
          tunnel: w385 -> [w389 w392]
          tunnel: w384 -> [w388 w391]
          tunnel: [w387 w390] -> w383
          frame "Ground", Default {
            n207 = call "GroundPassWrapper.vi"("State"=w389, "error in"=w388) -> ("error out"=w387:errorcluster)  [unwired: 9 in]
          }
          frame "Elevated" {
            n208 = call "ElevatedPass.vi"("PassState"=w392, "error in (no error)"=w391) -> ("error out"=w390:errorcluster)  [unwired: 9 in]
          }
        }
      }
    }
    n209 = Wait (ms)(milliseconds to wait=u32 50) -> ()  [unwired: 1 out]
    "PassIterations" <- w370
  }
  n210 = while {
    tunnel: [w404] -> _
    tunnel: "error in" -> [w398]
    i -> [w402]
    stop <- FALSE stop-if-true
    # "LowGoalShot"
    n211 = global read "Robot Global Data.vi" "cLowGoalShot"() -> (w394:bool)
    n212 = call "LoopTime.vi"() -> ("LoopTime"=→"LowGoalShotTimer":u32)  [unwired: 11 in]
    n213 = call "CheckButtonPressed.vi"("error in (no error)"=w398, "Button"=w394) -> ("error out"=w400:errorcluster, "Pressed?"=w396:bool)  [unwired: 8 in]
    n214 = call "HandleLowGoal.vi"("InitState"=LowGoalState."Stop", "error in"=w400, "Toggle?"=w396) -> ("error out"=w399:errorcluster, "ShootState"=w393:T26)  [unwired: 7 in]
    n215 = case shown="True" w396 {
      tunnel: w399 -> [w405 w408]
      tunnel: [w405 w407] -> w404
      tunnel: w393 -> [_ w406]
      frame False {
      }
      frame True {
        n216 = call "LowGoalWrapper.vi"("State"=w406, "error in"=w408) -> ("error out"=w407:errorcluster)  [unwired: 9 in]
      }
    }
    n217 = Wait (ms)(milliseconds to wait=u32 50) -> ()  [unwired: 1 out]
    "LowGoalShotIterations" <- w402
  }
